vi "Cleanup.vi"(0 "Path Group in":refnum<class "Path Group.lvclass">, 11 "error in (no error)":errorcluster) -> (4 "Path Group out":refnum<class "Path Group.lvclass">, 15 "error out":errorcluster)   [LabVIEW 2023, in "RFCalAndFixtureCharact.Common.lvlib" / "Path Group.lvclass"]
uses:
  Path Group.lvclass
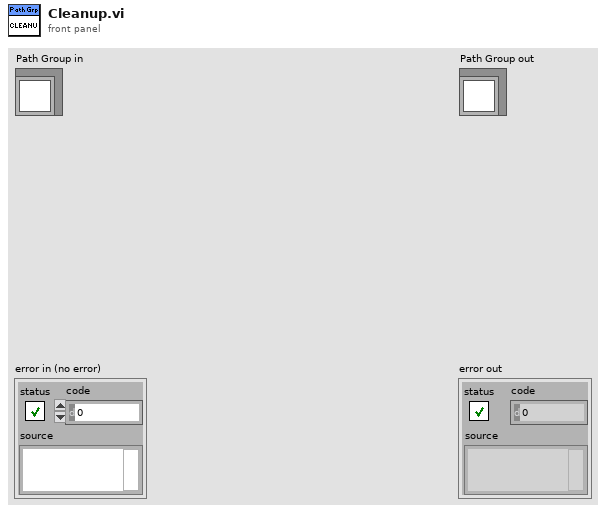
[diagram p1: front panel]
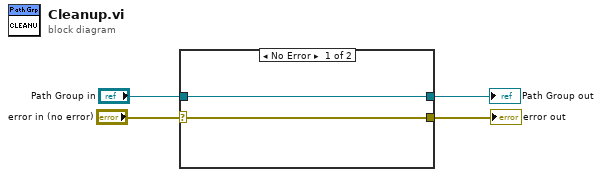
[diagram p0: block diagram]
diagram:
  n1 = case shown="No Error" "error in (no error)" {
    selector: "error in (no error)" -> [w5 w8]
    tunnel: [w5 w8] -> w3
    tunnel: [w6 w7] -> w1
    tunnel: "Path Group in" -> [w6 w7]
    frame No Error {
    }
    frame Error {
    }
  }
  "error out" <- w3
  "Path Group out" <- w1
